vi "python_지도 열기.vi"() -> ()   [LabVIEW 2023]
panel:
  in  "WebBrowser":refnum<k7>(container) caption="웹 브라우저"
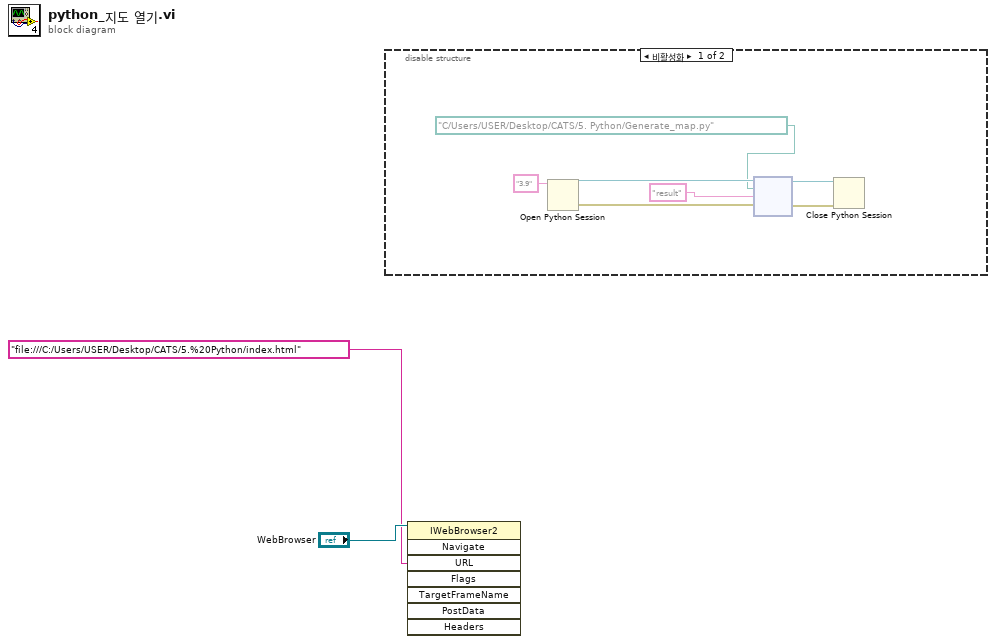
[diagram p0: block diagram]
diagram:
  n1 = disable-structure shown="비활성화" {
    frame Disabled {
      n2 = Open Python Session(python version="3.9" ("Python 버전")) -> (session out=w4:refnum<k35>, error out=w8:errorcluster)  [unwired: 2 in]
      n3 = node(w4, path "C:/Users/USER/Desktop/CATS/5. Python/Generate_map.py" ("모듈 경로"), "result" ("함수 이름"), w8) -> (w6:refnum<k35>, w5:errorcluster)  [unwired: 2 in, 2 out]
      n4 = Close Python Session(session in=w6, error in=w5) -> ()  [unwired: 1 out]
    }
    frame Enabled {
    }
  }
  n5 = invoke class="IWebBrowser2" method="Navigate"(reference="WebBrowser", "URL"="file:///C:/Users/USER/Desktop/CATS/5.%20Python/index.html" ("url")) -> ()  [unwired: 6 in, 8 out]
